vi "sound.vi"() -> ()   [LabVIEW 2015]
uses:
  <vilib>/NXT/Block Support/NXT_InputPort.ctl
  <vilib>/NXT/Subs/MotorOutput.ctl
  <vilib>/NXT/Dual Mode Library/Sensors/Sound_dB.vi
  <vilib>/NXT/Dual Mode Library/Motors/MotorOn.vi
panel:
  in  "Output Port (All Ports)":T1=3 items=["Port A", "Port B", "Port C", "All Ports"]
  in  "Port (Port 2)":T2=1 items=["Port 1", "Port 2", "Port 3", "Port 4"]
  out "웨이브폼 차트":i16(graph)
  in  "stop":bool
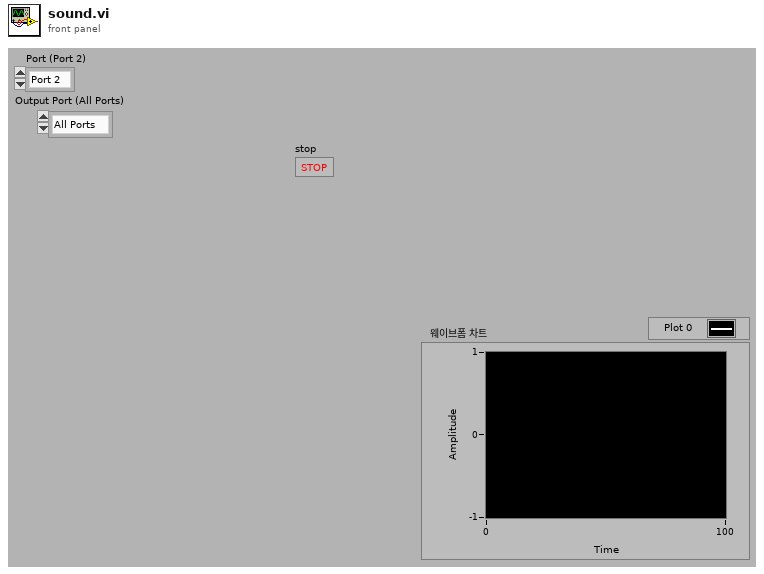
[diagram p1: front panel]
types:
  T1 = typedef "MotorOutput.ctl" = u8
  T2 = typedef "NXT_InputPort.ctl" = u32
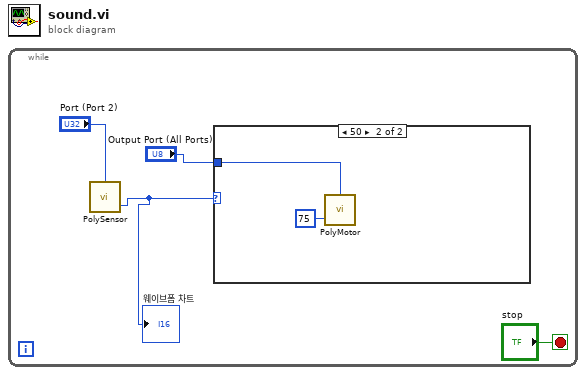
[diagram p0: block diagram]
diagram:
  n1 = while {
    stop <- "stop" stop-if-true
    n2 = call-poly <vilib>:"PolySensor.vi"("Port (Port 2)"="Port (Port 2)") -> ("Sound (dB)"=w2:i16)  [unwired: 2 in, 1 out]
    "웨이브폼 차트" <- w2
    n3 = case shown="50" w2 {
      tunnel: "Output Port (All Ports)" -> [_ w5]
      frame 0, Default {
      }
      frame 50 {
        n4 = call-poly <vilib>:"PolyMotor.vi"("Power (75)"=75, "Output Port (All Ports)"=w5) -> ()  [unwired: 2 in, 1 out]
      }
    }
  }
